vi "Clear Table.vi"(8 "error in (no error)":errorcluster, 11 "stats in":refnum<class "stats.lvclass">) -> (0 "error out":errorcluster, 3 "stats out":refnum<class "stats.lvclass">)   [LabVIEW 2012, in "stats.lvclass"]
uses:
  stats.lvclass
  stats.lvclass/stats.ctl
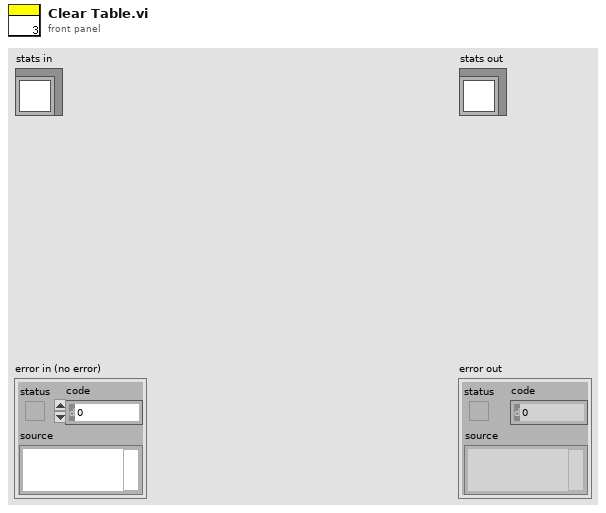
[diagram p1: front panel]
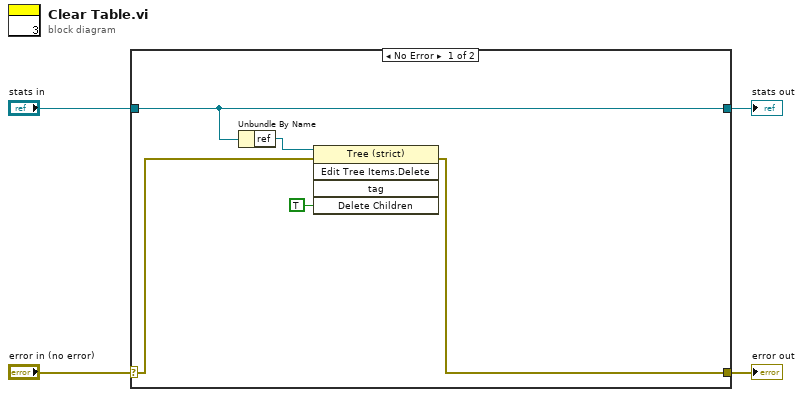
[diagram p0: block diagram]
diagram:
  n1 = case shown="No Error" "error in (no error)" {
    selector: "error in (no error)" -> [w6 w11]
    tunnel: [w5 w11] -> w3
    tunnel: [w9 w10] -> w1
    tunnel: "stats in" -> [w9 w10]
    frame No Error {
      n2 = Unbundle By Name(w9) -> ("ref"=w8:refnum<vi>)
      n3 = invoke class="Tree (strict)" method="Edit Tree Items.Delete"(reference=w8, error in=w6, "Delete Children"=TRUE ("Delete Children?")) -> (error out=w5:errorcluster)  [unwired: 2 in, 4 out]
    }
    frame Error {
    }
  }
  "error out" <- w3
  "stats out" <- w1
